vi "ex1.vi"() -> ()   [LabVIEW 2017]
uses:
  <vilib>/regexp/Match Regular Expression.xnode
panel:
  out "Array":string[](array[string])
  in  "Text":string
  in  "Letter":string
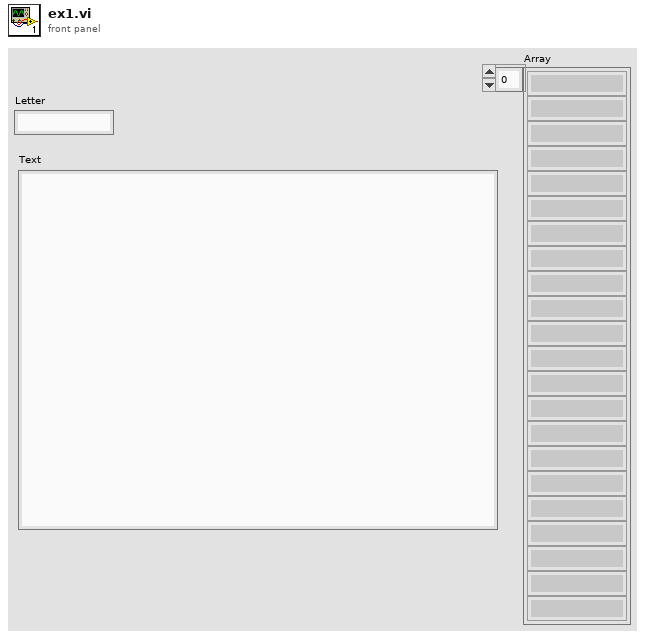
[diagram p1: front panel]
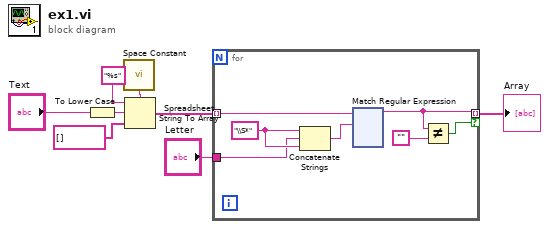
[diagram p0: block diagram]
diagram:
  n1 = To Lower Case(string="Text") -> (all lower case string=w6:string)
  n2 = call <vilib>:"Space Constant.vi"() -> ("String"=w1:string)
  n3 = Spreadsheet String To Array(delimiter (Tab)=w1, format string="%s", spreadsheet string=w6, array type (2D Dbl)=string[] []) -> (array=w4:string[])
  n4 = for {
    tunnel: w4 -> [w14] mode=indexing
    tunnel: "Letter" -> [w12]
    tunnel: [w10] -> w2 mode=indexing if=w15
    w13 = "\\S*" ("string")
    n5 = Concatenate Strings(w13, w12, w13) -> (w11:string)
    n6 = xnode "Match Regular Expression"("input string"=w14, "regular expression"=w11) -> ("whole match"=w10:string)  [unwired: 4 in, 4 out]
    n7 = Not Equal?(x=w10, y="") -> (x != y?=w15:bool)
  }
  "Array" <- w2
